vi "ep_Delay Integral Samples.vi"(8 "state in":dbl[](array[numeric]), 10 "delay":i32, 11 "signal in":dbl[](array[numeric])) -> (0 "state out":dbl[](array[numeric]), 3 "signal out":dbl[](array[numeric]))   [LabVIEW 2014, in "NI_EP_Motor Monitoring.lvlib"]
uses:
  <vilib>/addons/Electrical Power/Motor Monitoring/NI_EP_Motor Monitoring.lvlib
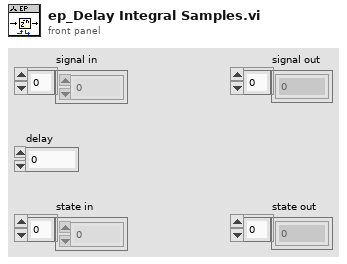
[diagram p1: front panel]
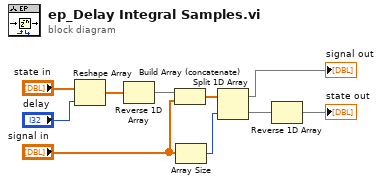
[diagram p0: block diagram]
diagram:
  n1 = Reshape Array("state in", "delay") -> (w10:dbl[])
  n2 = Reverse 1D Array(array=w10) -> (reversed array=w9:dbl[])
  n3 = Build Array (concatenate)(w9, "signal in") -> (w8:dbl[])
  n4 = Array Size(array="signal in") -> (size(s)=w6:i32)
  n5 = Split 1D Array(array=w8, index=w6) -> (first subarray=→"signal out":dbl[], second subarray=w7:dbl[])
  n6 = Reverse 1D Array(array=w7) -> (reversed array=→"state out":dbl[])
